vi "Configure Comparator Sequence.vi"(8 "error in (no error)":errorcluster, 10 "Limit Values Array":dbl[](array[numeric])=[0.0, 0.0, 0.0, 0.0, 0.0], 11 "VISA resource name":refnum<visa-resource-name>) -> (0 "error out":errorcluster, 3 "VISA resource name out":refnum<visa-resource-name>)   [LabVIEW 2016, in "Agilent E4980.lvlib"]
doc: "Sets the low and high limit values of the BINs for the comparator function in sequential mode.\n\n<B>Notes:</B>\n(1) The limit values are valid only when you select the limit mode as sequential. \n\n(2) The lower limit value must be lower than that of the upper limit value."
uses:
  <instrlib>/Agilent E4980/Agilent E4980.lvlib
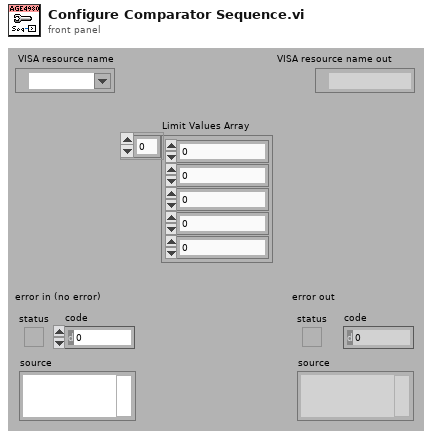
[diagram p1: front panel]
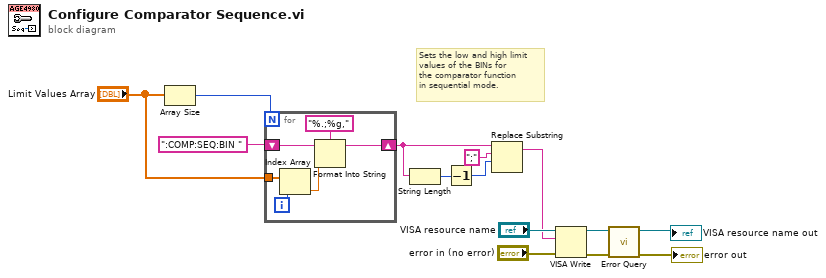
[diagram p0: block diagram]
diagram:
  # "Sets the low and high limit\nvalues of the BINs for\nthe comparator function\nin sequential mode."
  n1 = Array Size(array="Limit Values Array") -> (size(s)=w1:i32)
  n2 = for {
    N: w1 -> [_]
    shift-right: [w15] -> w13
    shift-left: ":COMP:SEQ:BIN " -> [w19]
    tunnel: "Limit Values Array" -> [w18]
    i -> [w17]
    n3 = Index Array(array=w18, index=w17) -> (element=w16:dbl)
    n4 = Format Into String(format string="%.;%g,", initial string=w19, w16) -> (resulting string=w15:string)  [unwired: 1 in, 1 out]
  }
  n5 = String Length(string=w13) -> (length=w12:i32)
  n6 = Decrement(x=w12) -> (x-1=w11:i32)
  n7 = Replace Substring(3:w11, 4:";" ("substring (\"\")"), 5:w13) -> (1:w7:string)  [unwired: 1 in, 1 out]
  n8 = VISA Write(VISA resource name="VISA resource name", write buffer=w7, error in (no error)="error in (no error)") -> (VISA resource name out=w6:refnum<visa-resource-name>, error out=w5:errorcluster)  [unwired: 1 out]
  n9 = call <instrlib>:"Error Query.vi"("error in (no error)"=w5, "VISA resource name"=w6) -> ("error out"=→"error out":errorcluster, "VISA resource name out"=→"VISA resource name out":refnum<visa-resource-name>)  [unwired: 6 in, 2 out]
